vi "Funktionsgenerator.vi"() -> ()   [LabVIEW 2017]
uses:
  <vilib>/Utility/error.llb/DialogType.ctl
  <vilib>/Analysis/3filter.llb/Filter Passband Type.ctl
  <vilib>/DAQmx/read.llb/DAQmx Read (Analog Wfm 1Chan NSamp).vi
  <vilib>/DAQmx/create/channels.llb/DAQmx Create Channel (AI-Voltage-Basic).vi
  <vilib>/DAQmx/configure/timing.llb/DAQmx Timing (Sample Clock).vi
  <vilib>/DAQmx/miscellaneous.llb/DAQmx Fill In Error Info.vi
  <vilib>/Analysis/3filter.llb/Chebyshev Filter (DBL).vi
  <vilib>/express/express analysis/Spectral/Block/exnSpectralBlock spectral measurements power poly.vi
  <vilib>/express/express analysis/Spectral/Block/exnSpectralBlock spectral measurements power WFM.vi
  <vilib>/Analysis/3filter.llb/Butterworth Filter (DBL).vi
  <vilib>/Utility/file.llb/Write Delimited Spreadsheet (DBL).vi
  <vilib>/express/express analysis/Spectral/XNode/ExpressSpectralMeasurementsBlockNode.xnode
  <vilib>/Analysis/NI_AALBase.lvlib
panel:
  in  "Abschneidefrequenz":dbl=0.12500000000000006 format="%0.4f"
  in  "Signalart":enum16{"AM Signal", "PM Signal", "FM Signal"}(ring)
  in  "Angenommene Trägerfrequenz":dbl
  in  "Speichern":bool
  out "Spektrum\nEingang":cluster{"f0":dbl, "df":dbl, "magnitude":dbl[]}(graph)
  out "Spektrum nach\nDemodulation":cluster{"f0":dbl, "df":dbl, "magnitude":dbl[]}(graph)
  out "Nach Demodulation":waveform(dbl)(graph)
  out "Eingang":waveform(dbl)(graph)
  in  "Demodulator":T1(ring)
  out "Spektrum nach Tiefpass":cluster{"f0":dbl, "df":dbl, "magnitude":dbl[]}(graph)
  in  "stop":bool
  out "Nach Tiefpass":waveform(dbl)(graph)
  in  "Niedrigster Wert":dbl=-10.0 format="%0.2f"
  in  "Höchster Wert":dbl=10.0 format="%0.2f"
  in  "Rate":dbl=40000.0 format="%0.2f"
  in  "Eingangskanal":tag="Dev3/ai0"
  in  "Zahl d. Datenpunkte":i32=4000
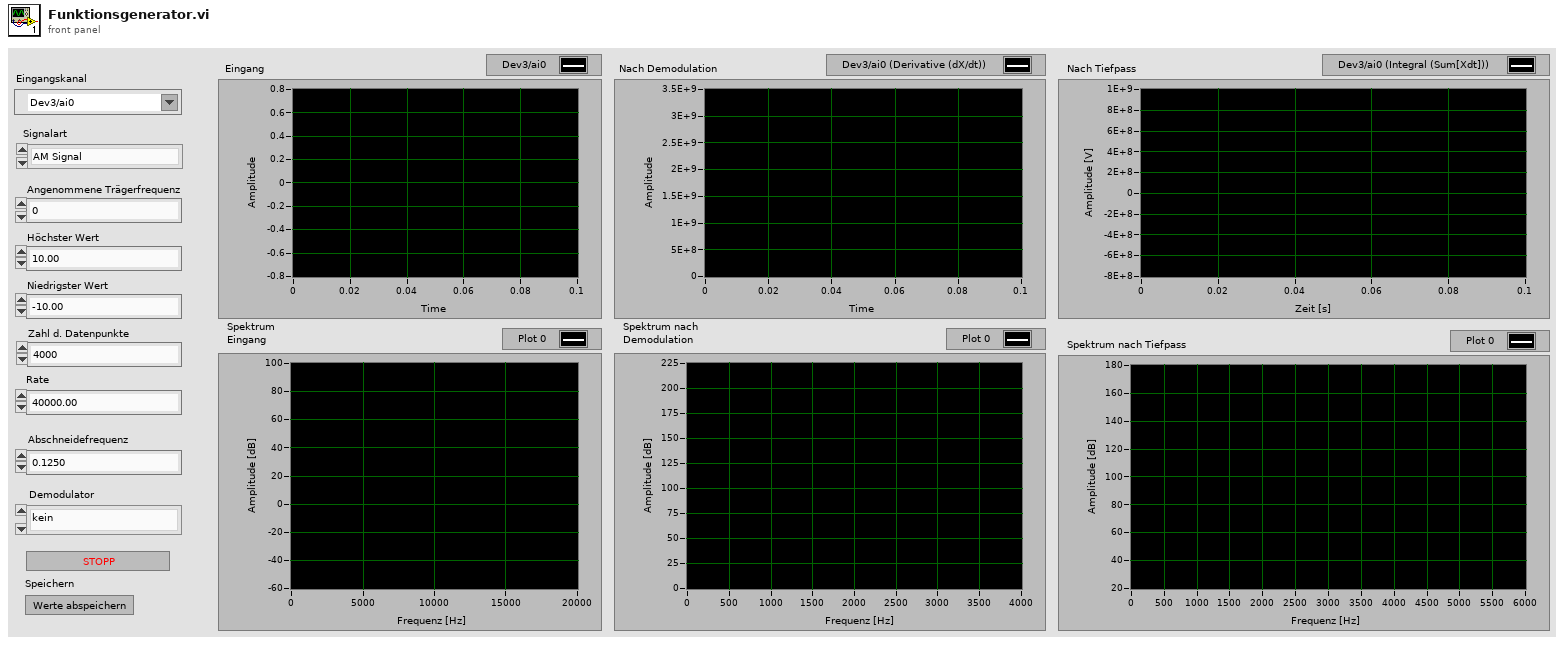
[diagram p1: front panel]
types:
  T1 = enum16{"kein", "Multiplikation mit Träger", "Quadrat", "Betrag"}
  T2 = typedef "NI_AALBase.lvlib/Filter Passband Type.ctl" = enum32{"Lowpass", "Highpass", "Bandpass", "Bandstop"}
  T3 = cluster{"averaging mode":u16, "weighting mode":u16, "number of averages":u32}
  T4 = cluster{"dB On (F)":bool, "unwrap phase (F)":bool, "convert to degree (F)":bool}
  T5 = typedef "DialogType.ctl" = u16
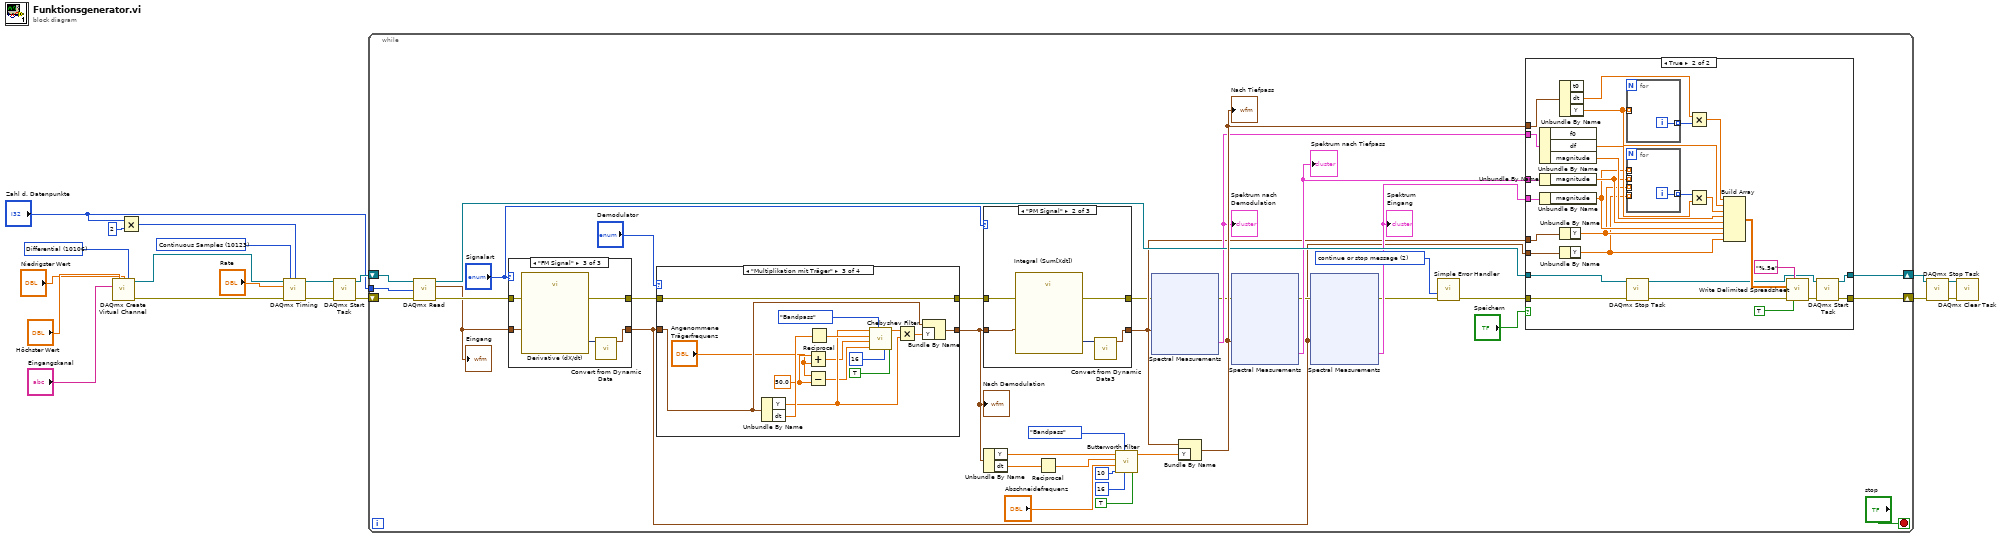
[diagram p0: block diagram]
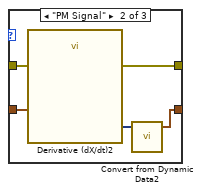
[diagram p5: hidden frame]
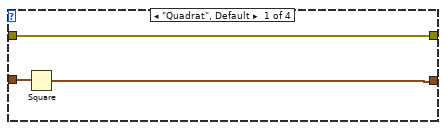
[diagram p7: hidden frame]
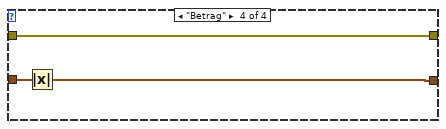
[diagram p9: hidden frame]
diagram:
  w5 = 10123 items=["Finite Samples"=10178, "Continuous Samples"=10123, "Hardware Timed Single Point"=12522] ("sample mode")
  w3 = 10106 items=["Default"=-1, "RSE"=10083, "NRSE"=10078, "Differential"=10106, "Pseudodifferential"=12529] ("input terminal configuration")
  n1 = call-poly <vilib>:"DAQmx Create Virtual Channel.vi"("maximum value"="Höchster Wert", "minimum value"="Niedrigster Wert", "input terminal configuration"=w3, "physical channels"="Eingangskanal") -> ("task out"=w14:refnum<k21>, "error out"=w19:errorcluster)  [unwired: 10 in]
  n2 = Multiply(x="Zahl d. Datenpunkte", y=2 ("x*y")) -> (x*y=w2:i32)
  n3 = call-poly <vilib>:"DAQmx Timing.vi"("task/channels in"=w14, "sample mode"=w5, "samples per channel"=w2, "rate"="Rate", "error in"=w19) -> ("task out"=w13:refnum<k21>, "error out"=w18:errorcluster)  [unwired: 9 in]
  n4 = call <vilib>:"DAQmx Start Task.vi"("task/channels in"=w13, "error in"=w18) -> ("task out"=w12:refnum<k21>, "error out"=w17:errorcluster)  [unwired: 12 in]
  n5 = while {
    shift-right: [w36] -> w16
    shift-left: w17 -> [w55]
    shift-right: [w37] -> w11
    shift-left: w12 -> [w54]
    tunnel: "Zahl d. Datenpunkte" -> [w52]
    stop <- "stop" stop-if-true
    w51 = T5 2 items=["no dialog", "OK message", "continue or stop message", "OK message + warnings", "continue/stop + warnings"] ("type of dialog (OK msg:1)")
    n6 = call-poly <vilib>:"DAQmx Read.vi"("task/channels in"=w54, "number of samples per channel"=w52, "error in"=w55) -> ("task out"=w38:refnum<k21>, "data"=w26:waveform(dbl), "error out"=w29:errorcluster)  [unwired: 10 in]
    "Eingang" <- w26
    n7 = case shown="\"FM Signal\"" "Signalart" {
      tunnel: w26 -> [w66 w70 w76]
      tunnel: [w66 w67 w72] -> w27
      tunnel: w29 -> [w65 w71 w75]
      tunnel: [w65 w69 w74] -> w28
      frame "AM Signal" {
      }
      frame "PM Signal" {
        n8 = call "Derivative (dX/dt)2"("error in (no error)"=w71, "Signals"=w70) -> ("error out"=w69:errorcluster, "Result"=w68:dynamicdata)  [unwired: 4 in]
        n9 = call "Convert from Dynamic Data2"("Dynamic Data Type"=w68) -> ("Waveform"=w67:waveform(dbl))  [unwired: 3 in]
      }
      frame "FM Signal" {
        n10 = call "Derivative (dX/dt)"("error in (no error)"=w75, "Signals"=w76) -> ("error out"=w74:errorcluster, "Result"=w73:dynamicdata)  [unwired: 4 in]
        n11 = call "Convert from Dynamic Data"("Dynamic Data Type"=w73) -> ("Waveform"=w72:waveform(dbl))  [unwired: 3 in]
      }
    }
    n12 = case shown="\"Multiplikation mit Träger\"" "Demodulator" {
      tunnel: w27 -> [w129 w131 w136 w149]
      tunnel: [w128 w131 w141 w148] -> w24
      tunnel: w28 -> [w127 w130 w140 w147]
      tunnel: [w127 w130 w140 w147] -> w23
      frame "Quadrat", Default {
        n13 = Square(x=w129) -> (x^2=w128:waveform(dbl))
      }
      frame "kein" {
      }
      frame "Multiplikation mit Träger" {
        w134 = 50.0 ("x")
        n14 = Unbundle By Name(w136) -> ("Y"=w138:dbl[], "dt"=w142:dbl)
        n15 = Add(x=w134, y="Angenommene Trägerfrequenz") -> (x+y=w135:dbl)
        n16 = Subtract(x="Angenommene Trägerfrequenz", y=w134) -> (x-y=w132:dbl)
        n17 = Reciprocal(x=w142) -> (1/x=w144:dbl)
        n18 = call-poly <vilib>:"Chebyshev Filter.vi"("init/cont (init:F)"=TRUE, "order"=16, "filter type"=Filter_Passband_Type."Bandpass", "low cutoff freq: fl"=w132, "high cutoff freq: fh"=w135, "sampling freq: fs"=w144, "X"=w138) -> ("Filtered X"=w139:dbl[])  [unwired: 3 in, 1 out]
        n19 = Multiply(x=w139, y=w138) -> (x*y=w137:dbl[])
        n20 = Bundle By Name(cluster=w136, "Y"=w137) -> (w141:waveform(dbl))
      }
      frame "Betrag" {
        n21 = Absolute Value(x=w149) -> (abs(x)=w148:waveform(dbl))
      }
    }
    "Nach Demodulation" <- w24
    n22 = case shown="\"PM Signal\"" "Signalart" {
      tunnel: w24 -> [w57 w62 w64]
      tunnel: w23 -> [w56 w61 w63]
      tunnel: [w56 w60 w63] -> w21
      tunnel: [w57 w58 w64] -> w22
      frame "AM Signal", Default {
      }
      frame "PM Signal" {
        n23 = call "Integral (Sum[Xdt])"("error in (no error)"=w61, "Signals"=w62) -> ("error out"=w60:errorcluster, "Result"=w59:dynamicdata)  [unwired: 4 in]
        n24 = call "Convert from Dynamic Data3"("Dynamic Data Type"=w59) -> ("Waveform"=w58:waveform(dbl))  [unwired: 3 in]
      }
      frame "FM Signal" {
      }
    }
    n25 = Unbundle By Name(w24) -> ("Y"=w47:dbl[], "dt"=w42:dbl)
    n26 = Reciprocal(x=w42) -> (1/x=w46:dbl)
    n27 = call-poly <vilib>:"Butterworth Filter.vi"("init/cont (init:F)"=TRUE, "order"=16, "filter type"=Filter_Passband_Type."Bandpass", "low cutoff freq: fl"=i16 10, "high cutoff freq: fh"="Abschneidefrequenz", "sampling freq: fs"=w46, "X"=w47) -> ("Filtered X"=w43:dbl[])  [unwired: 1 in, 1 out]
    n28 = xnode "Spectral Measurements"("Signals"=w22, "error in (no error)"=w21) -> ("Power Spectrum"=w34:cluster{"f0":dbl, "df":dbl, "magnitude":dbl[]}, "error out"=w32:errorcluster)
    "Spektrum nach\nDemodulation" <- w34
    n29 = Bundle By Name(cluster=w22, "Y"=w43) -> (w40:waveform(dbl))
    "Nach Tiefpass" <- w40
    n30 = xnode "Spectral Measurements"("Signals"=w40, "error in (no error)"=w32) -> ("Power Spectrum"=w35:cluster{"f0":dbl, "df":dbl, "magnitude":dbl[]}, "error out"=w31:errorcluster)
    "Spektrum nach Tiefpass" <- w35
    n31 = xnode "Spectral Measurements"("Signals"=w27, "error in (no error)"=w31) -> ("Power Spectrum"=w33:cluster{"f0":dbl, "df":dbl, "magnitude":dbl[]}, "error out"=w30:errorcluster)
    "Spektrum\nEingang" <- w33
    n32 = call <vilib>:"Simple Error Handler.vi"("type of dialog (OK msg:1)"=w51, "error in (no error)"=w30) -> ("error out"=w39:errorcluster)  [unwired: 3 in, 4 out]
    n33 = case shown="True" "Speichern" {
      tunnel: w38 -> [w78 w95]
      tunnel: [w78 w89] -> w37
      tunnel: w39 -> [w77 w93]
      tunnel: [w77 w90] -> w36
      tunnel: w35 -> [_ w87]
      tunnel: w40 -> [_ w86]
      tunnel: w34 -> [_ w88]
      tunnel: w33 -> [_ w84]
      tunnel: w22 -> [_ w82]
      tunnel: w27 -> [_ w81]
      frame False {
      }
      frame True {
        n34 = Unbundle By Name(w88) -> ("df"=w100:dbl, "magnitude"=w104:dbl[])  [unwired: 1 out]
        n35 = Unbundle By Name(w87) -> ("magnitude"=w98:dbl[])
        n36 = Unbundle By Name(w84) -> ("magnitude"=w85:dbl[])
        n37 = Unbundle By Name(w86) -> ("dt"=w102:dbl, "Y"=w96:dbl[])  [unwired: 1 out]
        n38 = Unbundle By Name(w82) -> ("Y"=w80:dbl[])
        n39 = Unbundle By Name(w81) -> ("Y"=w79:dbl[])
        n40 = for {
          tunnel: [w108] -> w99 mode=indexing
          tunnel: w96 -> [_] mode=indexing
          i -> [w108]
        }
        n41 = for {
          tunnel: w98 -> [_] mode=indexing
          tunnel: [w107] -> w83 mode=indexing
          tunnel: w85 -> [_] mode=indexing
          tunnel: w80 -> [_] mode=indexing
          tunnel: w79 -> [_] mode=indexing
          i -> [w107]
        }
        n42 = call <vilib>:"DAQmx Stop Task.vi"("task/channels in"=w95, "error in"=w93) -> ("task out"=w94:refnum<k21>, "error out"=w92:errorcluster)  [unwired: 12 in]
        n43 = Multiply(x=w102, y=w99) -> (x*y=w101:dbl[])
        n44 = Multiply(x=w83, y=w100) -> (x*y=w97:dbl[])
        n45 = Build Array(w101, w96, w97, w104, w98, w85, w80, w79) -> (w103:dbl[][])
        n46 = call-poly <vilib>:"Write Delimited Spreadsheet.vi"("format (%.3f)"="%.5e", "2D data"=w103, "error in (no error)"=w92, "transpose? (no:F)"=TRUE) -> ("error out"=w91:errorcluster)  [unwired: 10 in, 1 out]
        n47 = call <vilib>:"DAQmx Start Task.vi"("task/channels in"=w94, "error in"=w91) -> ("task out"=w89:refnum<k21>, "error out"=w90:errorcluster)  [unwired: 12 in]
      }
    }
  }
  n48 = call <vilib>:"DAQmx Stop Task.vi"("task/channels in"=w11, "error in"=w16) -> ("task out"=w10:refnum<k21>, "error out"=w15:errorcluster)  [unwired: 12 in]
  n49 = call <vilib>:"DAQmx Clear Task.vi"("task in"=w10, "error in"=w15) -> ()  [unwired: 13 in, 1 out]
